vi "UDP roboRIO recieve.vi"(8 "error in (no error)":errorcluster, 9 "ENQUE DIRECTLY":refnum<queue>, 10 "milliseconds to wait":u32, 11 "UDP Network Connection in":refnum<k16>) -> (0 "error out":errorcluster)   [LabVIEW 2016]
uses:
  Globale Variablen VI/RadSensoren.vi
panel:
  out "data out":string
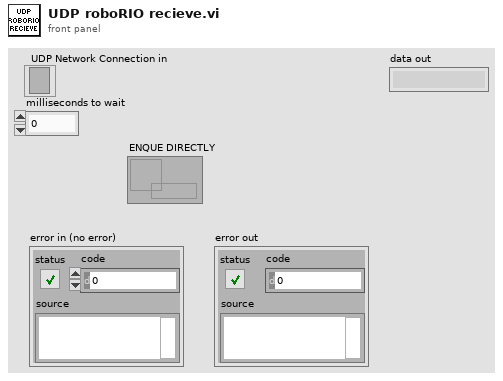
[diagram p1: front panel]
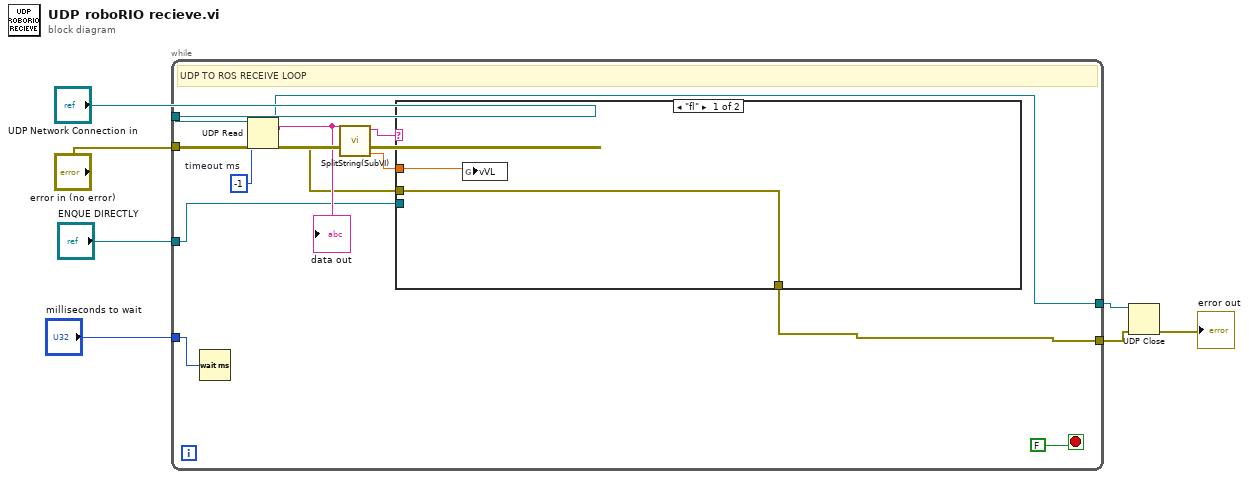
[diagram p0: block diagram]
diagram:
  n1 = while {
    tunnel: [w16] -> w6
    tunnel: "UDP Network Connection in" -> [w18]
    tunnel: "error in (no error)" -> [w17]
    tunnel: "milliseconds to wait" -> [w12]
    tunnel: [w8] -> w2
    tunnel: "ENQUE DIRECTLY" -> [w11]
    stop <- FALSE stop-if-true
    w19 = -1  # timeout ms
    # "UDP TO ROS RECEIVE LOOP"
    n2 = Wait (ms)(milliseconds to wait=w12) -> ()  [unwired: 1 out]
    n3 = UDP Read(connection ID=w18, timeout ms (25000)=w19, 8:w17) -> (data out=w13:string, error out=w10:errorcluster, 3:w16:refnum<k16>)  [unwired: 3 out]
    "data out" <- w13
    n4 = call "SplitString(SubVI).vi"("data in"=w13) -> ("Numeric"=w15:dbl, "String 3"=w14:string)  [unwired: 9 in]
    n5 = case shown="\"fl\"" w14 {
      tunnel: w15 -> [w21 _]
      tunnel: w10 -> [w20 w22]
      tunnel: [w20 w22] -> w8
      tunnel: w11 -> [_ _]
      frame "fl" {
        n6 = global write "RadSensoren.vi" "vVL"(w21) -> ()
      }
      frame Default {
      }
    }
  }
  n7 = UDP Close(connection ID=w6, 8:w2) -> (error out=→"error out":errorcluster)  [unwired: 1 out]
